vi "Apollo Compass Real.vi"(9 "Compass Com Port":refnum<visa-resource-name>, 10 "Compass In":dbl) -> (3 "Compass Out":dbl)   [LabVIEW 2014]
panel:
  # "Apollo Compass Real\nmar 28 2017"
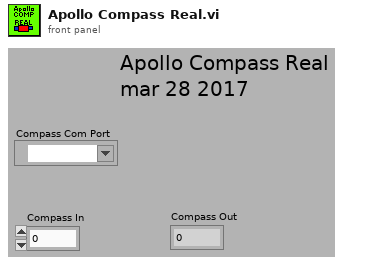
[diagram p1: front panel]
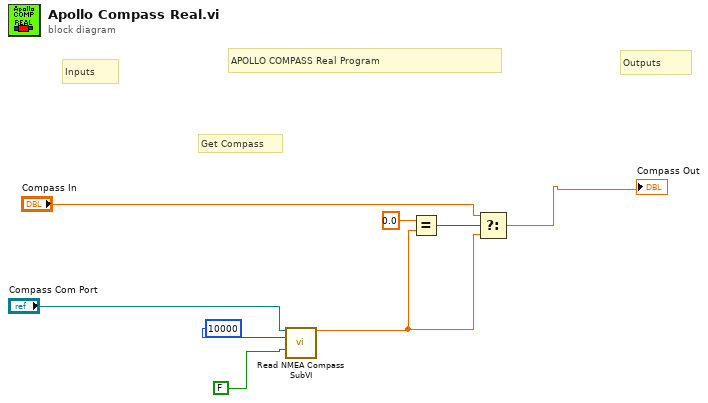
[diagram p0: block diagram]
diagram:
  # "Get Compass"
  # "APOLLO COMPASS Real Program"
  # "Outputs"
  # "Inputs"
  n1 = call "Read NMEA Compass SubVI.vi"("VISA resource name"="Compass Com Port", "timeout (ms)"=u32 10000 ("time out"), "stop"=FALSE) -> ("Heading"=w1:dbl)  [unwired: 10 in, 2 out]
  n2 = Equal?(x=0.0, y=w1) -> (x = y?=w2:bool)
  n3 = Select(t="Compass In", s=w2, f=w1) -> (s? t:f=→"Compass Out":dbl)
